vi "Asylum_GetLabel.vi"(8 "error in (no error)":errorcluster, 10 "parameterName":string, 11 "Application":refnum<k7>) -> (0 "error out":errorcluster, 2 "Label":string, 3 "Application":refnum<k7>)   [LabVIEW 2019]
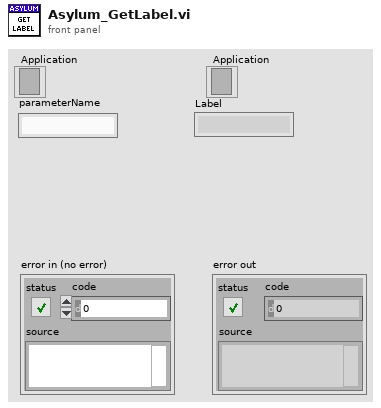
[diagram p1: front panel]
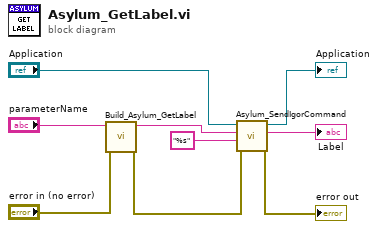
[diagram p0: block diagram]
diagram:
  n1 = call "Build_Asylum_GetLabel.vi"("error in (no error)"="error in (no error)", "parameterName"="parameterName") -> ("error out"=w9:errorcluster, "Command"=w7:string)  [unwired: 8 in]
  n2 = call "Asylum_SendIgorCommand.vi"("error in (no error)"=w9, "Format"="%s", "command"=w7, "Application In"="Application") -> ("error out"=→"error out":errorcluster, "results"=→"Label":string, "Application Out"=→"Application":refnum<k7>)  [unwired: 4 in, 1 out]
